vi "Called.vi"() -> ()   [LabVIEW 2020]
panel:
  out "error out":errorcluster
  in  "error in (no error)":errorcluster
  in  "Back":bool
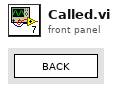
[diagram p1: front panel]
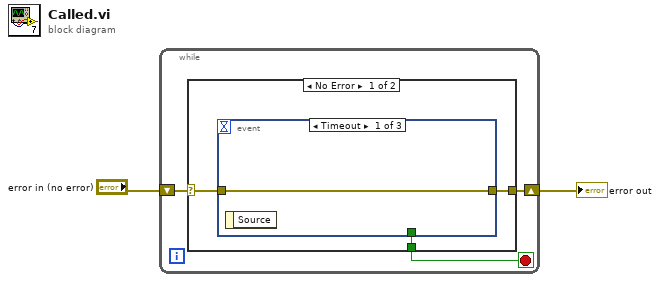
[diagram p0: block diagram]
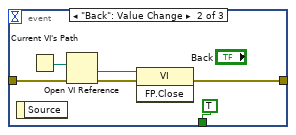
[diagram p2: hidden frame]
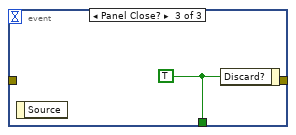
[diagram p3: hidden frame]
diagram:
  n1 = while {
    shift-right: [w4] -> w1
    shift-left: "error in (no error)" -> [w5]
    stop <- w3 stop-if-true
    n2 = case shown="No Error" w5 {
      selector: w5 -> [w8 w17]
      tunnel: [w7 w17] -> w4
      tunnel: [w6 _] -> w3
      frame No Error {
        n3 = event shown="[0] Timeout" {
          selector: _ -> [_ _ _]
          dyn-events: _ -> [_ _ _]
          timeout: _ -> [_ _ _]
          tunnel: [w9 w12 _] -> w7
          tunnel: w8 -> [w9 w11 _]
          tunnel: [_ TRUE ("Discard?") w16] -> w6
          event Timeout {
            n4 = event-data() -> ()  [unwired: 1 in, 1 out]
          }
          event "Back": Value Change {
            n5 = event-data() -> ()  [unwired: 1 in, 1 out]
            n6 = Current VI's Path() -> (path=w15:path)
            n7 = Open VI Reference(vi path=w15, error in (no error)=w11) -> (vi reference=w14:refnum<vi>, error out=w13:errorcluster)  [unwired: 4 in]
            n8 = invoke class="VI" method="FP.Close"(reference=w14, error in=w13) -> (error out=w12:errorcluster)  [unwired: 1 in, 2 out]
          }
          event Panel Close? {
            w16 = TRUE ("Discard?")
            n9 = event-data() -> ()  [unwired: 1 in, 1 out]
            n10 = event-data("Discard?"=w16) -> ()  [unwired: 1 in, 1 out]
          }
        }
      }
      frame Error {
      }
    }
  }
  "error out" <- w1
